vi "Create Data OD reference.vi"(8 "error in (no error)":errorcluster, 11 "Experiment in":refnum<class "Experiment.lvclass">) -> (0 "error out":errorcluster, 3 "Experiment out":refnum<class "Experiment.lvclass">)   [LabVIEW 2020, in "Experiment.lvclass"]
uses:
  Experiment.lvclass
  Experiment.lvclass/Experiment.ctl
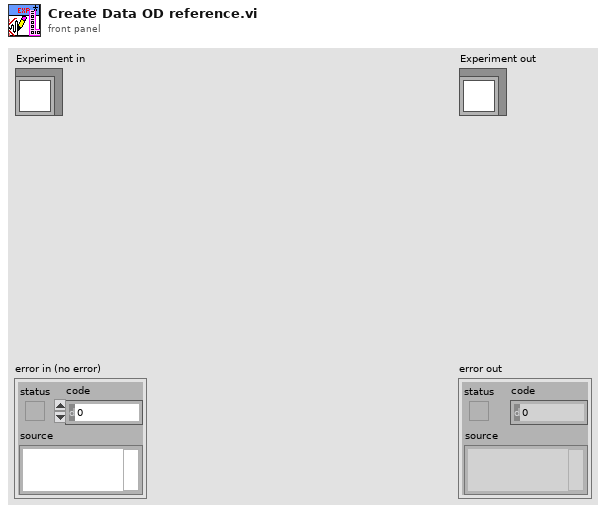
[diagram p1: front panel]
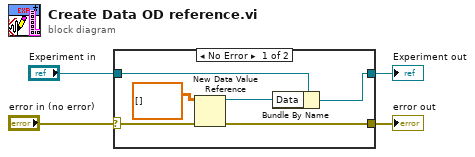
[diagram p0: block diagram]
diagram:
  n1 = case shown="No Error" "error in (no error)" {
    selector: "error in (no error)" -> [w9 w11]
    tunnel: [w8 w11] -> w3
    tunnel: [w10 w12] -> w1
    tunnel: "Experiment in" -> [w6 w12]
    frame No Error {
      n2 = New Data Value Reference(data value=sgl[][] [] ("initialized array"), error in=w9) -> (data value reference=w5:refnum<data-value>, error out=w8:errorcluster)
      n3 = Bundle By Name(cluster=w6, "Data"=w5) -> (w10:refnum<class "Experiment.lvclass">)
    }
    frame Error {
    }
  }
  "error out" <- w3
  "Experiment out" <- w1
